vi "Heat2D_Form X RHS.vi"(4 "Matr_RHS":dbl[][](array[numeric]), 6 "step":i32, 7 "U(n)":dbl[][](array[numeric]), 8 "Boundary Condition":cluster{"type":T2, "Value":dbl[][]}[](array[cluster]) {"type" items=["Dirichlet", "Neumann"]}, 9 "X RHS":dbl[][](array[numeric]), 10 "Coefficients":T1={"rx"=0.0, "ry"=0.0, "s"=-0.0, "c"=0.0, "deltaT"=0.0, "deltaX"=0.0, "deltaY"=0.0}, 11 "F(t, x, y)":dbl[][][](array[numeric])=array1x101x101[10201 elements]) -> (1 "X RHS out":dbl[][](array[numeric]), 2 "U(M)":dbl[](array[numeric]), 3 "U(0)":dbl[](array[numeric]))   [LabVIEW 2020, in "NI_PDE.lvlib"]
uses:
  <vilib>/gmath/NI_PDE.lvlib
  <vilib>/gmath/pde.llb/Common/PDE_BC Type.ctl
  <vilib>/Analysis/2dsp.llb/2D Convolution (DBL).vi
  <vilib>/Analysis/NI_AALPro.lvlib
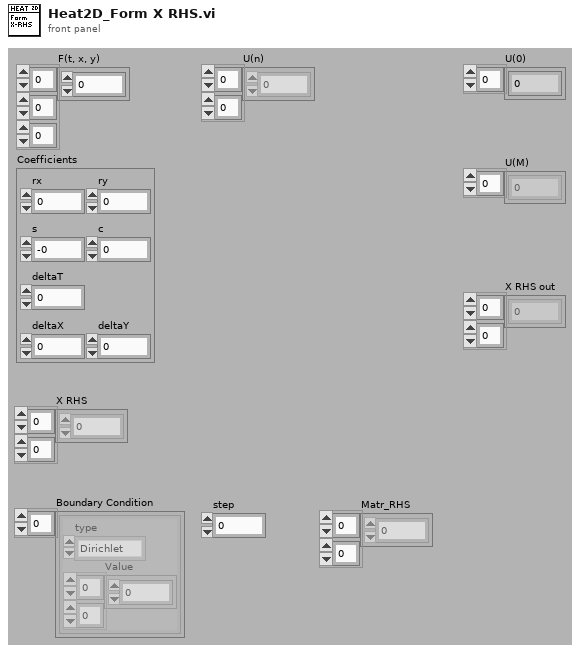
[diagram p1: front panel]
types:
  T1 = cluster{"rx":dbl, "ry":dbl, "s":dbl, "c":dbl, "deltaT":dbl, "deltaX":dbl, "deltaY":dbl}
  T2 = typedef "NI_PDE.lvlib/PDE_BC Type.ctl" = i32
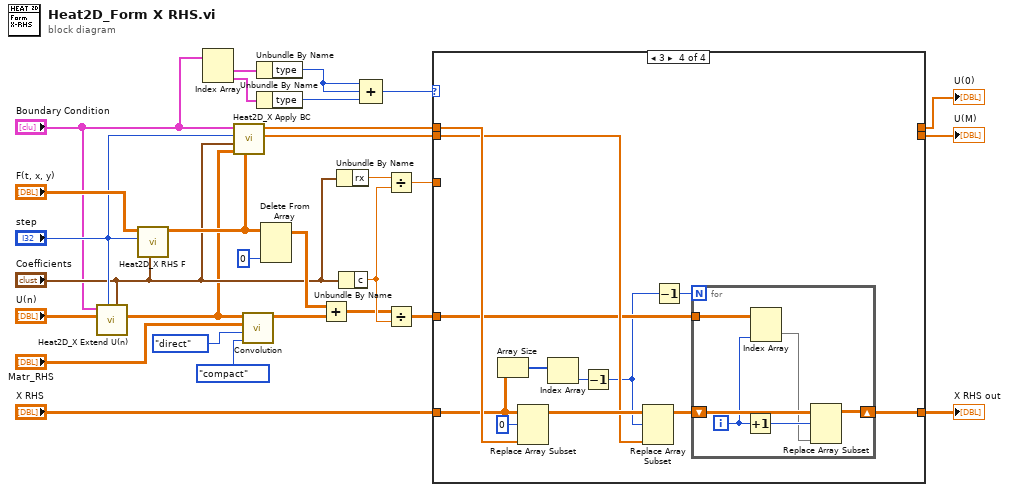
[diagram p0: block diagram]
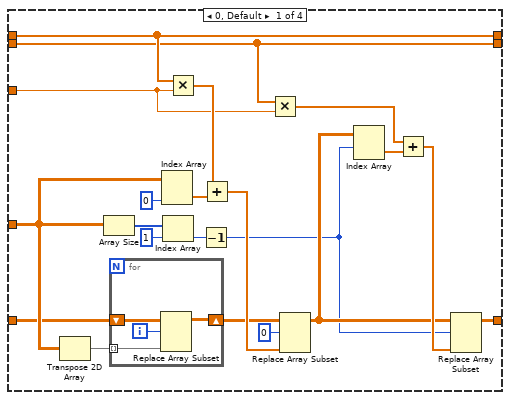
[diagram p2: hidden frame]
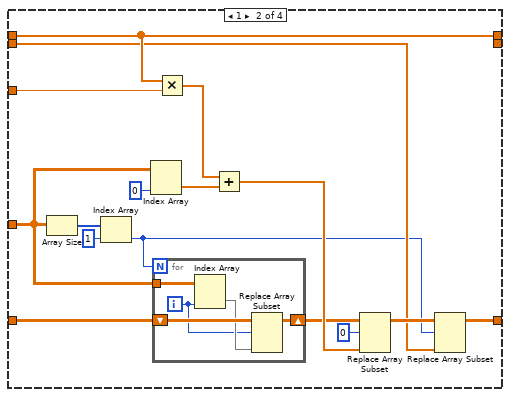
[diagram p3: hidden frame]
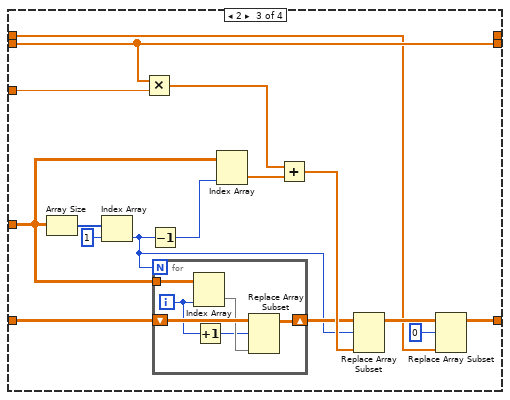
[diagram p4: hidden frame]
diagram:
  n1 = call <vilib>:"Heat2D_X Extend U(n).vi"("Coefficients"="Coefficients", "step"="step", "U(n)"="U(n)", "Boundary Condition"="Boundary Condition") -> ("Interp(X)"=w1:dbl[][])  [unwired: 3 in, 4 out]
  n2 = call <vilib>:"Heat2D_X RHS F.vi"("Coefficients"="Coefficients", "step"="step", "F(n+1)+F(n)"="F(t, x, y)") -> ("F"=w6:dbl[][])  [unwired: 8 out]
  n3 = Index Array(array="Boundary Condition") -> (element #1=w29:cluster{"type":T2, "Value":dbl[][]}, element #2=w28:cluster{"type":T2, "Value":dbl[][]})  [unwired: 2 in]
  n4 = call <vilib>:"Heat2D_X Apply BC.vi"("F(n+1)+F(n)"=w6, "Extended U(n)"=w1, "Coefficients"="Coefficients", "step"="step", "Boundary Condition"="Boundary Condition") -> ("U Right"=w9:dbl[], "U Left"=w8:dbl[])  [unwired: 5 out]
  n5 = call-poly <vilib>:"Convolution.vi"("output size"=enum32{"full", "size X", "compact"}."compact", "algorithm"=enum32{"direct", "frequency domain"}."direct", "Y"="Matr_RHS", "X"=w1) -> ("X * Y"=w19:dbl[][])  [unwired: 7 out]
  n6 = Unbundle By Name(w29) -> ("type"=w27:T2)
  n7 = Unbundle By Name(w28) -> ("type"=w26:T2)
  n8 = Delete From Array(array=w6, index (col)=0 ("disabled index (col)")) -> (array with subset deleted=w20:dbl[][])  [unwired: 2 in, 1 out]
  n9 = Add(x=w20, y=w19) -> (x+y=w18:dbl[][])
  n10 = Unbundle By Name("Coefficients") -> ("rx"=w25:dbl)
  n11 = Unbundle By Name("Coefficients") -> ("c"=w24:dbl)
  n12 = Compound Arithmetic op=ADD(w27, w27, w26) -> (w15:T2)
  n13 = Divide(x=w25, y=w24) -> (x/y=w16:dbl)
  n14 = Divide(x=w18, y=w24) -> (x/y=w13:dbl[][])
  n15 = case shown="3" w15 {
    tunnel: w13 -> [w31 w59 w83 w102]
    tunnel: [w39 w62 w77 w101] -> w10
    tunnel: w8 -> [w48 w68 w78 w108]
    tunnel: w9 -> [w45 w61 w91 w106]
    tunnel: [w48 w68 _ _] -> w12
    tunnel: [w45 _ w91 _] -> w11
    tunnel: w16 -> [w46 w69 w90 _]
    tunnel: "X RHS" -> [w30 w55 w76 w98]
    frame 0, Default {
      n16 = Transpose 2D Array(2D array=w31) -> (transposed array=w32:dbl[][])
      n17 = Array Size(array=w31) -> (size(s)=w43:i32[])
      n18 = for {
        shift-right: [w53] -> w34
        shift-left: w30 -> [w54]
        tunnel: w32 -> [w51] mode=indexing
        i -> [w52]
        n19 = Replace Array Subset(array=w54, new element=w51, index (row)=w52) -> (w53:dbl[][])  [unwired: 1 in]
      }
      n20 = Index Array(array=w31, index (col)=0 ("disabled index (col)")) -> (element=w49:dbl[])  [unwired: 1 in]
      n21 = Index Array(array=w43, index=1) -> (element=w33:i32)
      n22 = Multiply(x=w48, y=w46) -> (x*y=w47:dbl[])
      n23 = Decrement(x=w33) -> (x-1=w35:i32)
      n24 = Add(x=w47, y=w49) -> (x+y=w42:dbl[])
      n25 = Multiply(x=w45, y=w46) -> (x*y=w44:dbl[])
      n26 = Replace Array Subset(array=w34, new element=w42, index (row)=0) -> (w38:dbl[][])  [unwired: 1 in]
      n27 = Index Array(array=w38, index (row)=w35) -> (element=w50:dbl[])  [unwired: 1 in]
      n28 = Add(x=w44, y=w50) -> (x+y=w41:dbl[])
      n29 = Replace Array Subset(array=w38, new element=w41, index (row)=w35) -> (w39:dbl[][])  [unwired: 1 in]
    }
    frame 1 {
      n30 = Array Size(array=w59) -> (size(s)=w58:i32[])
      n31 = Index Array(array=w58, index=1) -> (element=w56:i32)
      n32 = Index Array(array=w59, index (col)=0 ("disabled index (col)")) -> (element=w70:dbl[])  [unwired: 1 in]
      n33 = for {
        N: w56 -> [_]
        shift-right: [w71] -> w60
        shift-left: w55 -> [w74]
        tunnel: w59 -> [w75]
        i -> [w72]
        n34 = Index Array(array=w75, index (col)=w72) -> (element=w73:dbl[])  [unwired: 1 in]
        n35 = Replace Array Subset(array=w74, new element=w73, index (row)=w72) -> (w71:dbl[][])  [unwired: 1 in]
      }
      n36 = Multiply(x=w68, y=w69) -> (x*y=w67:dbl[])
      n37 = Add(x=w67, y=w70) -> (x+y=w65:dbl[])
      n38 = Replace Array Subset(array=w60, new element=w65, index (row)=0) -> (w66:dbl[][])  [unwired: 1 in]
      n39 = Replace Array Subset(array=w66, new element=w61, index (row)=w56) -> (w62:dbl[][])  [unwired: 1 in]
    }
    frame 2 {
      n40 = Array Size(array=w83) -> (size(s)=w89:i32[])
      n41 = Index Array(array=w89, index=1) -> (element=w81:i32)
      n42 = Multiply(x=w91, y=w90) -> (x*y=w84:dbl[])
      n43 = Decrement(x=w81) -> (x-1=w86:i32)
      n44 = for {
        N: w81 -> [_]
        shift-right: [w92] -> w82
        shift-left: w76 -> [w96]
        tunnel: w83 -> [w97]
        i -> [w94]
        n45 = Index Array(array=w97, index (col)=w94) -> (element=w95:dbl[])  [unwired: 1 in]
        n46 = Increment(x=w94) -> (x+1=w93:i32)
        n47 = Replace Array Subset(array=w96, new element=w95, index (row)=w93) -> (w92:dbl[][])  [unwired: 1 in]
      }
      n48 = Index Array(array=w83, index (col)=w86) -> (element=w85:dbl[])  [unwired: 1 in]
      n49 = Add(x=w84, y=w85) -> (x+y=w88:dbl[])
      n50 = Replace Array Subset(array=w82, new element=w88, index (row)=w81) -> (w80:dbl[][])  [unwired: 1 in]
      n51 = Replace Array Subset(array=w80, new element=w78, index (row)=0) -> (w77:dbl[][])  [unwired: 1 in]
    }
    frame 3 {
      n52 = Array Size(array=w98) -> (size(s)=w105:i32[])
      n53 = Replace Array Subset(array=w98, new element=w108, index (row)=0) -> (w107:dbl[][])  [unwired: 1 in]
      n54 = Index Array(array=w105) -> (element=w104:i32)  [unwired: 1 in]
      n55 = Decrement(x=w104) -> (x-1=w100:i32)
      n56 = Replace Array Subset(array=w107, new element=w106, index (row)=w100) -> (w103:dbl[][])  [unwired: 1 in]
      n57 = Decrement(x=w100) -> (x-1=w99:i32)
      n58 = for {
        N: w99 -> [_]
        shift-right: [w114] -> w101
        shift-left: w103 -> [w115]
        tunnel: w102 -> [w112]
        i -> [w111]
        n59 = Increment(x=w111) -> (x+1=w113:i32)
        n60 = Index Array(array=w112, index (col)=w111) -> (element=w110:dbl[])  [unwired: 1 in]
        n61 = Replace Array Subset(array=w115, new element=w110, index (row)=w113) -> (w114:dbl[][])  [unwired: 1 in]
      }
    }
  }
  "U(0)" <- w12
  "U(M)" <- w11
  "X RHS out" <- w10
